vi "Set Position Setpoint.vi"(8 "error in (no error)":errorcluster, 10 "CCW position (rad)":dbl, 11 "KUKA youBot arm motor_EtherCAT in":refnum<class "NI_Robotics_KUKA youBot Arm Motor_EtherCAT.lvclass">) -> (0 "error out":errorcluster, 3 "KUKA youBot arm motor_EtherCAT out":refnum<class "NI_Robotics_KUKA youBot Arm Motor_EtherCAT.lvclass">)   [LabVIEW 2017, in "NI_Robotics_KUKA youBot Host.lvlib" / "NI_Robotics_KUKA youBot Arm Motor_EtherCAT.lvclass"]
uses:
  <vilib>/robotics/KUKA youBot/Motor/Arm Motor EtherCAT/NI_Robotics_KUKA youBot Arm Motor_EtherCAT.lvclass
  c:/Program Files (x86)/National Instruments/LabVIEW 2017/vi.lib/robotics/KUKA youBot/Motor/Arm Motor/NI_Robotics_KUKA youBot Arm Motor.lvclass
  <vilib>/robotics/KUKA youBot/Motor/Arm Motor EtherCAT/NI_Robotics_KUKA youBot Arm Motor_EtherCAT.lvclass/NI_Robotics_KUKA youBot Arm Motor_EtherCAT.ctl
  <vilib>/robotics/KUKA youBot/Motor/Arm Motor/NI_Robotics_KUKA youBot Arm Motor.lvclass
  <vilib>/robotics/KUKA youBot/NI_Robotics_KUKA youBot Host.lvlib
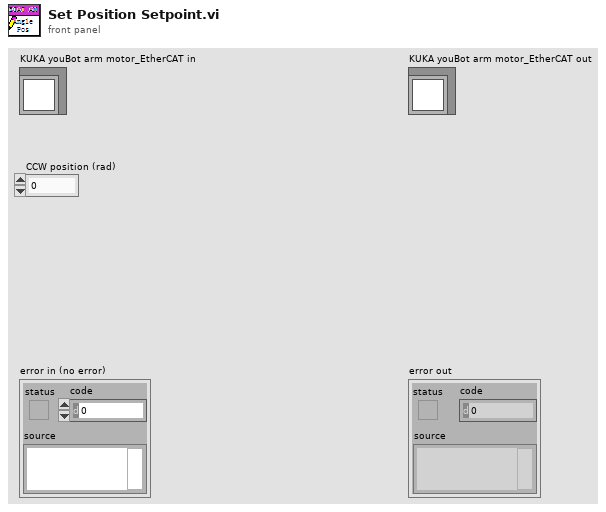
[diagram p1: front panel]
types:
  T1 = typedef "NI_Robotics_KUKA youBot Host.lvlib/Motor Slave Info.ctl" = cluster{"controller mode var":refnum<k21>, "reference var":refnum<k21>, "current var":refnum<k21>, "velocity var":refnum<k21>, "position var":refnum<k21>, "status var":refnum<k21>, "valid":bool, "status var type":enum16{"Int16", "Int32"}, "nodeAddr":u16, "masterHdl":T2}
  T2 = typedef "NI_Robotics_KUKA youBot Host.lvlib/Mater Handler.ctl" = i32
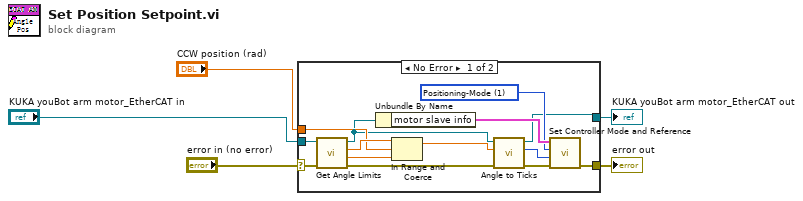
[diagram p0: block diagram]
diagram:
  n1 = case shown="No Error" "error in (no error)" {
    selector: "error in (no error)" -> [w18 w20]
    tunnel: "CCW position (rad)" -> [w15 _]
    tunnel: "KUKA youBot arm motor_EtherCAT in" -> [w19 w21]
    tunnel: [w14 w20] -> w2
    tunnel: [w7 w21] -> w1
    frame No Error {
      w12 = u8 1 items=["Motor Stop", "Positioning-Mode", "Velocity-Mode", "no more action", "set position to reference", "PWM-Mode", "Current-Mode", "Initialize"] ("controller mode")
      n2 = call <vilib>:"Get Angle Limits.vi"("error in (no error)"=w18, "KUKA youBot arm motor in"=w19) -> ("error out"=w11:errorcluster, "min angle (rad)"=w16:dbl, "max angle (rad)"=w17:dbl, "KUKA youBot arm motor out"=w8:refnum<class "NI_Robotics_KUKA youBot Arm Motor_EtherCAT.lvclass">)  [unwired: 6 in]
      n3 = Unbundle By Name(w8) -> ("motor slave info"=w13:T1)
      n4 = In Range and Coerce(upper limit=w17, x=w15, lower limit=w16) -> (coerced(x)=w9:dbl)  [unwired: 1 out]
      n5 = call <vilib>:"Angle to Ticks.vi"("error in (no error)"=w11, "angle (radian)"=w9, "KUKA youBot arm motor_EtherCAT in"=w8) -> ("error out"=w10:errorcluster, "ticks"=w6:i32, "KUKA youBot arm motor_EtherCAT out"=w7:refnum<class "NI_Robotics_KUKA youBot Arm Motor_EtherCAT.lvclass">)  [unwired: 6 in]
      n6 = call <vilib>:"Set Controller Mode and Reference.vi"("error in (no error)"=w10, "reference"=w6, "controller mode"=w12, "motor slave info in"=w13) -> ("error out"=w14:errorcluster)  [unwired: 5 in, 2 out]
    }
    frame Error {
    }
  }
  "error out" <- w2
  "KUKA youBot arm motor_EtherCAT out" <- w1
